vi "Register Sessions.vi"(8 "error in":errorcluster, 11 "request data":T2) -> (0 "error out":errorcluster, 3 "response data":T1)   [LabVIEW 2020, in "MeasurementLink Session Management Client Wrapper.lvlib"]
uses:
  MeasurementLink Session Management Client Wrapper.lvlib
  MeasurementLink Session Management Client/RPC Messages/ni_measurementlink_sessionmanagement_v1_RegisterSessionsRequest.ctl
  MeasurementLink Session Management Client/RPC Messages/ni_measurementlink_sessionmanagement_v1_SessionInformation.ctl
  MeasurementLink Session Management Client/RPC Messages/nidevice_grpc_Session.ctl
  MeasurementLink Session Management Client/RPC Messages/ni_measurementlink_sessionmanagement_v1_ChannelMapping.ctl
  MeasurementLink Session Management Client/RPC Messages/ni_measurementlink_sessionmanagement_v1_RegisterSessionsResponse.ctl
  Action.ctl
  MeasurementLink Session Management Client/MeasurementLink Session Management Client.lvlib
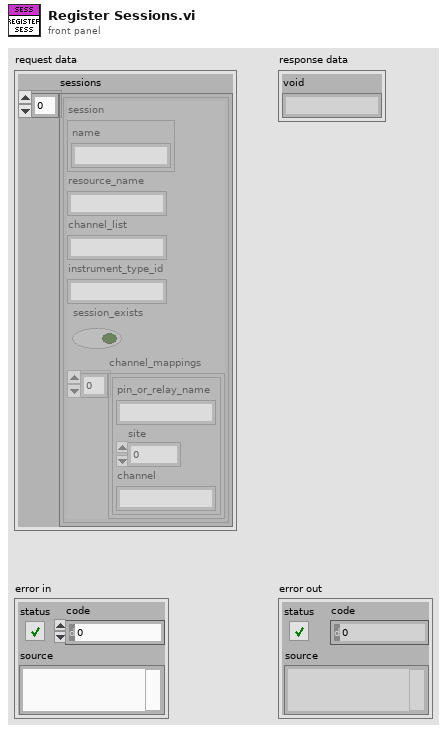
[diagram p1: front panel]
types:
  T1 = typedef "MeasurementLink Session Management Client.lvlib/ni_measurementlink_sessionmanagement_v1_RegisterSessionsResponse.ctl" = cluster{"void":string}
  T2 = typedef "MeasurementLink Session Management Client.lvlib/ni_measurementlink_sessionmanagement_v1_RegisterSessionsRequest.ctl" = cluster{"sessions":T3[]}
  T3 = typedef "MeasurementLink Session Management Client.lvlib/ni_measurementlink_sessionmanagement_v1_SessionInformation.ctl" = cluster{"session":T4, "resource_name":string, "channel_list":string, "instrument_type_id":string, "session_exists":bool, "channel_mappings":T5[]}
  T4 = typedef "MeasurementLink Session Management Client.lvlib/nidevice_grpc_Session.ctl" = cluster{"name":string}
  T5 = typedef "MeasurementLink Session Management Client.lvlib/ni_measurementlink_sessionmanagement_v1_ChannelMapping.ctl" = cluster{"pin_or_relay_name":string, "site":i32, "channel":string}
  T6 = typedef "MeasurementLink Session Management Client Wrapper.lvlib/Action.ctl" = enum16{"Get Client", "Destroy Client"}
  T7 = typedef "grpc-lvsupport-release.lvlib/grpcId.ctl" = u64
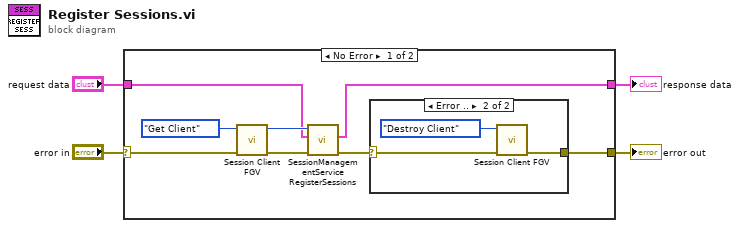
[diagram p0: block diagram]
diagram:
  n1 = case shown="No Error" "error in" {
    selector: "error in" -> [w12 w17]
    tunnel: [w8 w17] -> w3
    tunnel: "request data" -> [w6 _]
    tunnel: [w5 _] -> w1
    frame No Error {
      n2 = call "Session Client FGV.vi"("error in"=w12, "action"=Action."Get Client") -> ("error out"=w11:errorcluster, "grpc client id"=w10:T7)  [unwired: 8 in]
      n3 = call "SessionManagementService RegisterSessions.vi"("error in"=w11, "Request Data"=w6, "gRPC ID"=w10) -> ("error out"=w9:errorcluster, "Response Data"=w5:T1)  [unwired: 6 in, 1 out]
      n4 = case shown="Error .." w9 {
        selector: w9 -> [w13 w16]
        tunnel: [w13 w14] -> w8
        frame No Error {
        }
        frame Error {
          n5 = call "Session Client FGV.vi"("error in"=w16, "action"=Action."Destroy Client") -> ("error out"=w14:errorcluster)  [unwired: 8 in, 1 out]
        }
      }
    }
    frame Error {
    }
  }
  "error out" <- w3
  "response data" <- w1
